vi "FillianProj2.vi"() -> ()   [LabVIEW 2015]
uses:
  <vilib>/Utility/error.llb/Error Cluster From Error Code.vi
  <vilib>/ErrorRing/Error Ring.xnode
panel:
  out "Warnings 2":errorcluster
  out "Current Voltage":dbl(knob) scale=0.0..12.0
  out "Thermometer":dbl(slide) scale=0.0..30.0
  in  "Start/pause":bool
  out "?":bool
  out "?":bool
  out "?":bool
  out "?":bool
  out "?":bool
  out "?":bool
  out "?":bool
  out "?":bool
  out "?":bool
  out "?":bool
  out "?":bool
  out "?":bool
  out "?":bool
  out "?":bool
  out "?":bool
  out "?":bool
  out "Too high":bool
  out "Too low":bool
  out "Too cold":bool
  out "Too hot":bool
  in  "Max temp":sgl(slide) scale=20.0..45.0
  in  "Min temp":sgl(slide) scale=0.0..20.0
  in  "Min voltage":sgl(knob) min=0 max=12 step=0.5 scale=0.0..12.0
  in  "Max voltage":sgl(knob) min=0 max=12 step=0.5 scale=0.0..12.0
  out "Min":dbl(knob) scale=0.0..12.0
  out "Max":dbl(knob) scale=0.0..12.0
  out "Max":dbl(slide) scale=0.0..30.0
  out "Min":dbl(slide) scale=0.0..30.0
  out "Mean":dbl(slide) scale=0.0..30.0
  out "Mean":dbl(knob) scale=0.0..12.0
  out "Voltage":sgl(graph)
  out "Temperature":sgl(graph)
  out "Battery Timeout":bool
  out "Battery Timeout":bool
  out "Link Timeout":bool
  out "Link Timeout":bool
  out "Link Quality":sgl
  out "Battery Voltage":sgl
  out "Battery Voltage":sgl
  out "Link Quality":sgl
  in  "stop 2":bool
  # "Wireless Sensor Network Project"
  # "Temperature Sensor"
  # "Battery"
  # "Link quality"
  # "Voltage Sensor"
  # "Battery"
  # "Link quality"
  # "Warnings"
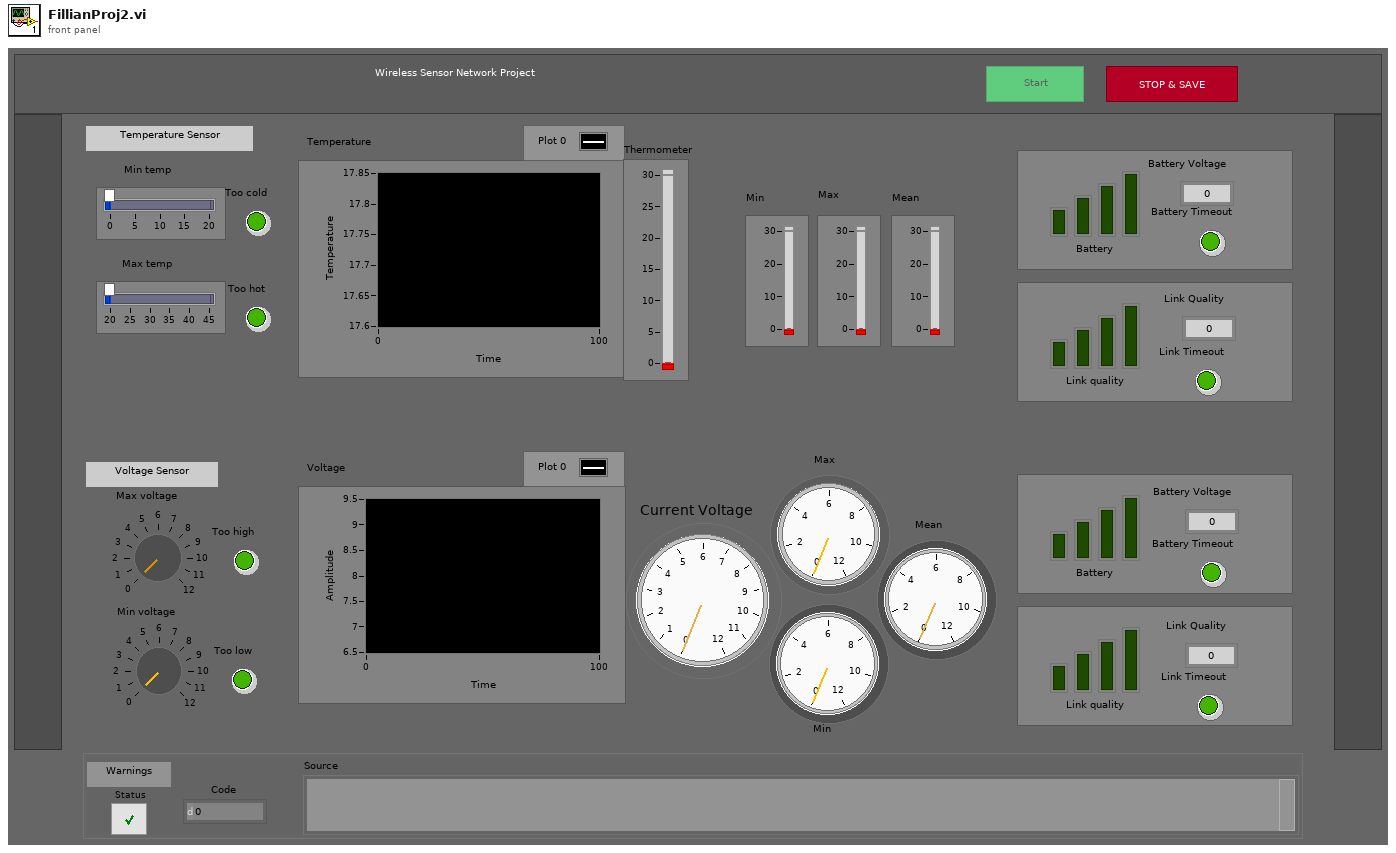
[diagram p1: front panel]
types:
  T1 = enum8{"Enabled", "Disabled", "Disabled and Grayed Out"}
  T2 = enum16{"open", "replace", "create", "open or create", "replace or create", "replace or create with confirmation"}
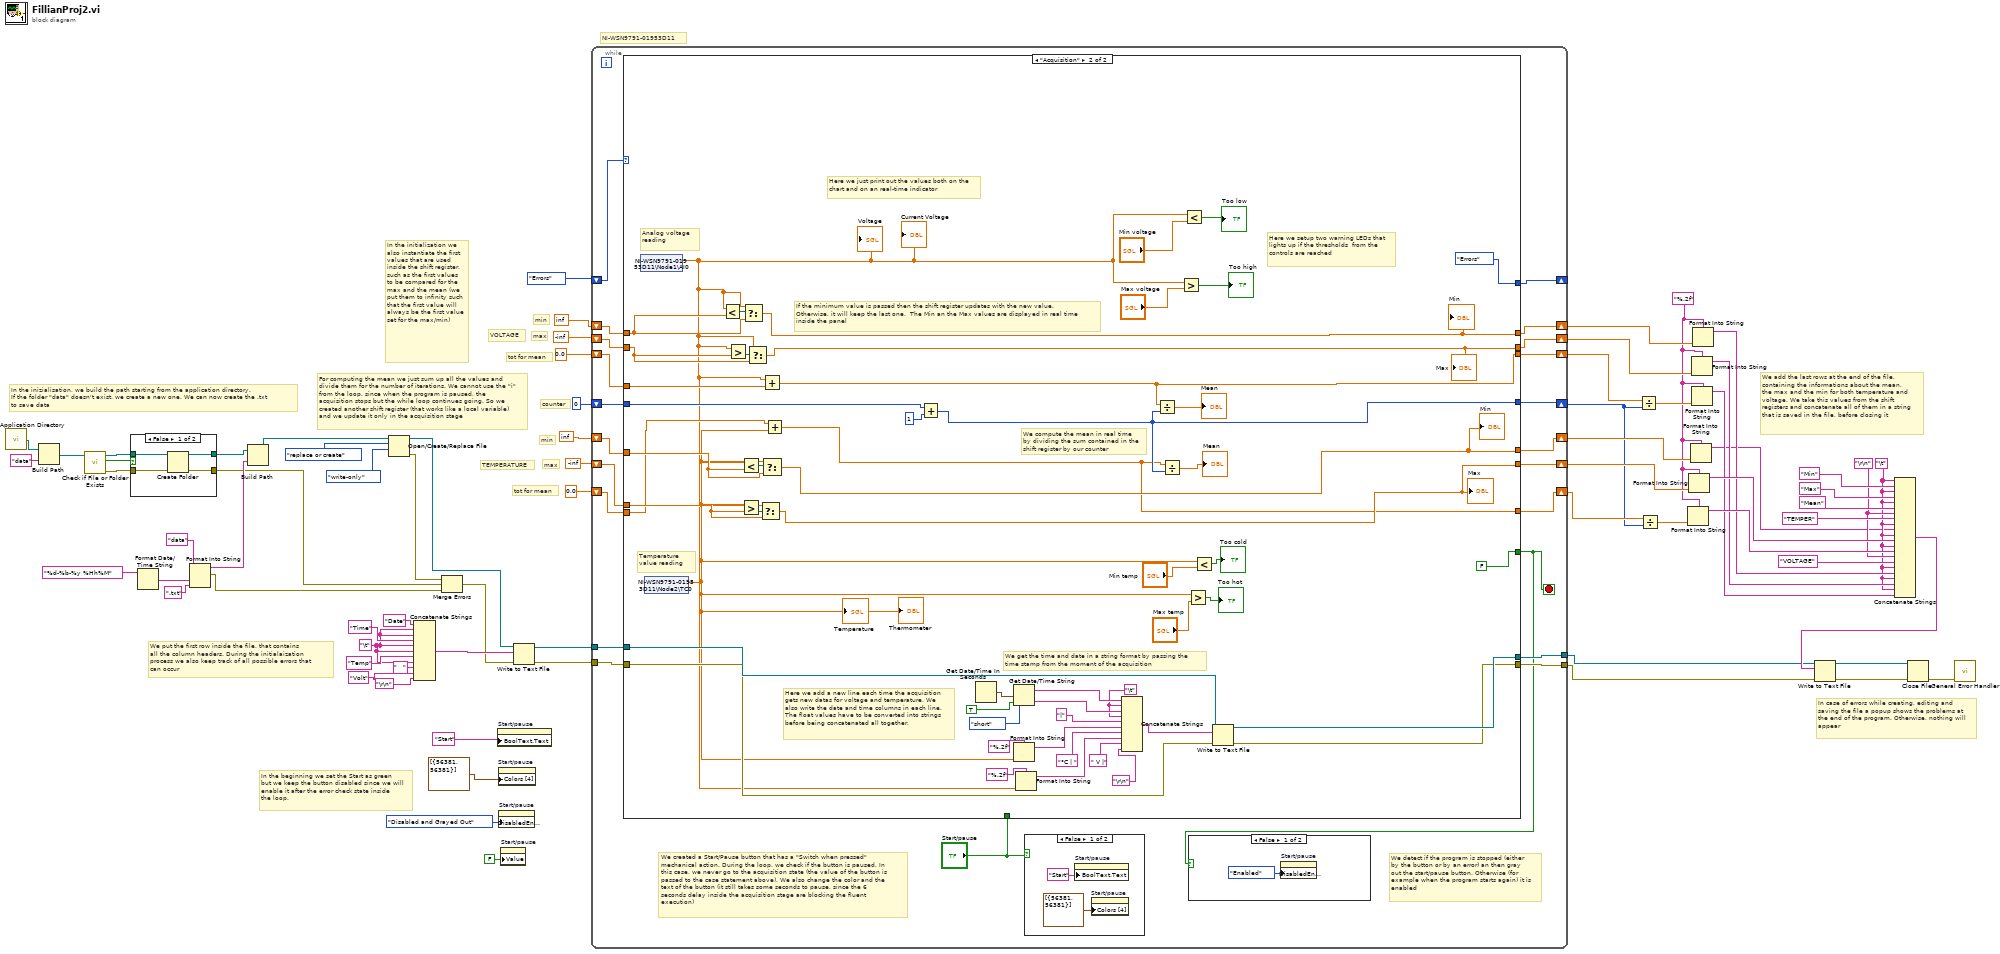
[diagram p0: block diagram]
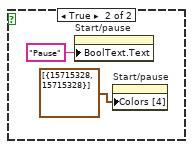
[diagram p3: hidden frame]
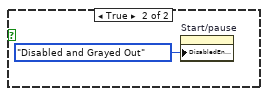
[diagram p4: hidden frame]
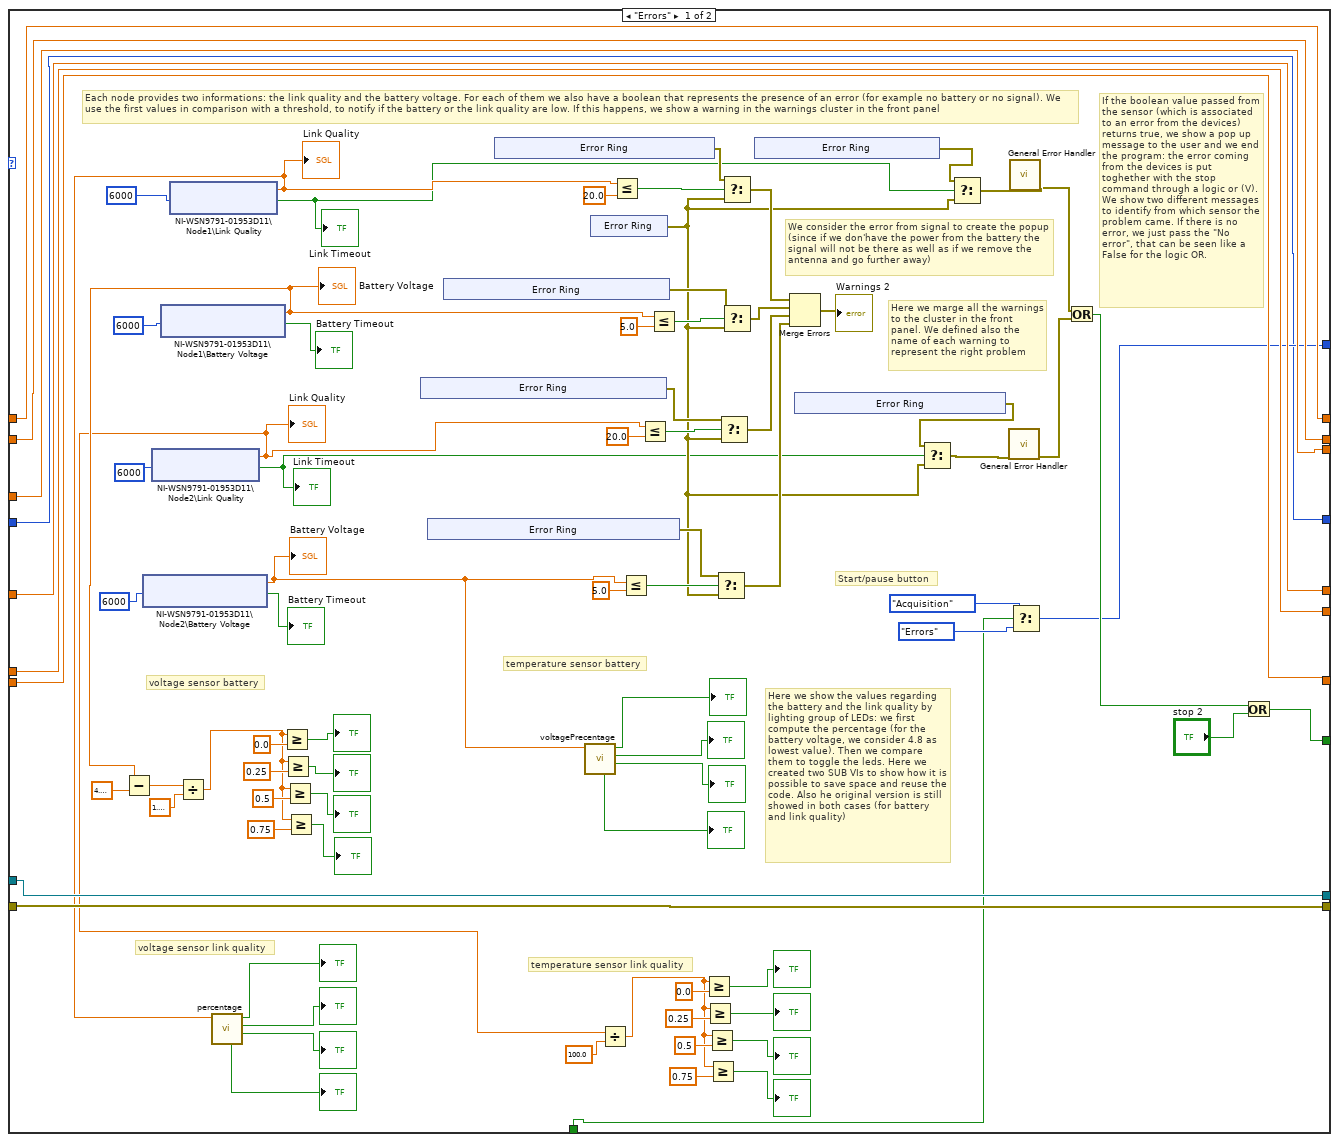
[diagram p5: hidden frame]
diagram:
  w5 = "%.2f" ("format string")
  w22 = "\t"
  w63 = "\r\n"
  w21 = "\t"
  # "We add the last rows at the end of the file, containing the informations about the mean, the max and the min for both temperature and voltage. We take this values from the shift registers and concatenate all of them in a string that is saved in the file, before closing it"
  # "In case of errors while creating, editing and saving the file a popup shows the problems at the end of the program. Otherwise, nothing will appear"
  # "In the beginning we set the Start as green but we keep the button disabled since we will enable it after the error check state inside the loop."
  # "In the initialization we also instantiate the first values that are used inside the shift register, such as the first values to be compared for the max and the mean (we put them to infinity such that the first value will always be the first value set for the max/min)"
  # "We put the first row inside the file, that contains\nall the column headers. During the initialaization \nprocess we also keep track of all possible errors that\ncan occur"
  # "In the inizialisation, we build the path starting from the application directory.\nIf the folder \"data\" doesn't exist, we create a new one. We can now create the .txt \nto save data"
  # "counter"
  # "For computing the mean we just sum up all the values and divide them for the number of iterations. We cannot use the \"i\" from the loop, since when the program is paused, the acquisition stops but the while loop continues going. So we created another shift register (that works like a local variable) and we update it only in the acquisition stage"
  # "NI-WSN9791-01953D11"
  # "max"
  # "tot for mean"
  # "min"
  # "max"
  # "tot for mean"
  # "min"
  # "VOLTAGE"
  # "TEMPERATURE"
  n1 = call <vilib>:"Application Directory.vi"() -> ("Application Directory"=w42:path)
  n2 = Build Path(base path=w42, name or relative path="data") -> (appended path=w40:path)
  n3 = call <vilib>:"Check if File or Folder Exists.vi"("path"=w40) -> ("error out"=w38:errorcluster, "file or folder exists?"=w37:bool, "dup path"=w39:path)  [unwired: 8 in]
  n4 = case shown="False" w37 {
    tunnel: w39 -> [w75 w77]
    tunnel: w38 -> [w74 w76]
    tunnel: [w73 w77] -> w36
    tunnel: [w72 w76] -> w28
    frame False {
      n5 = Create Folder(path (use dialog)=w75, error in=w74) -> (created path=w73:path, error out=w72:errorcluster)  [unwired: 1 in, 1 out]
    }
    frame True {
    }
  }
  n6 = Format Date/Time String(time format string (%c)="%d-%b-%y %Hh%M") -> (date/time string=w33:string)  [unwired: 2 in]
  n7 = Format Into String(initial string="data", w33, ".txt") -> (resulting string=w31:string, error out=w29:errorcluster)  [unwired: 2 in]
  n8 = Build Path(base path=w36, name or relative path=w31) -> (appended path=w30:path)
  n9 = Open/Create/Replace File(file path (use dialog)=w30, operation (0:open)=T2."replace or create", access (0:read/write)=enum16{"read/write", "read-only", "write-only"}."write-only") -> (refnum out=w11:refnum<file>, error out=w12:errorcluster)  [unwired: 3 in, 1 out]
  n10 = Concatenate Strings("Date" ("text"), w22, w22, "Time" ("text"), w22, w22, "Temp" ("text"), w22, "   " ("string"), "Volt" ("text"), "\r\n") -> (w50:string)
  n11 = Merge Errors(w12, w28, w29) -> (w27:errorcluster)
  n12 = property on="Start/pause" class="Bool (strict)"("BoolText.Text"="Start" ("Boolean Text.Text")) -> ()  [unwired: 2 in, 2 out]
  n13 = property on="Start/pause" class="Bool (strict)"("Colors [4]"=cluster{u32, u32}[] [{56381, 56381}]) -> ()  [unwired: 2 in, 2 out]
  n14 = property on="Start/pause" class="Bool (strict)"("DisabledEnum"=T1."Disabled and Grayed Out" ("Disabled")) -> ()  [unwired: 2 in, 2 out]
  n15 = property on="Start/pause" class="Bool (strict)"("Value"=FALSE ("Start/pause")) -> ()  [unwired: 2 in, 2 out]
  n16 = Write to Text File(file (use dialog)=w11, text=w50, error in=w27) -> (refnum out=w48:refnum<file>, error out=w47:errorcluster)  [unwired: 1 in, 1 out]
  n17 = while {
    shift-right: [w93] -> w56
    shift-left: inf -> [w99]
    shift-right: [w92] -> w55
    shift-left: -inf -> [w98]
    shift-right: [w91] -> w44
    shift-left: 0.0 -> [w97]
    shift-right: [w90] -> w54
    shift-left: inf -> [w96]
    shift-right: [w89] -> w53
    shift-left: -inf -> [w95]
    shift-right: [w88] -> w46
    shift-left: 0.0 -> [w94]
    tunnel: [w87] -> w3
    tunnel: [w86] -> w2
    tunnel: w48 -> [w85]
    tunnel: w47 -> [w84]
    shift-right: [w82] -> _
    shift-left: enum16{"Errors", "Acquisition"}."Errors" -> [w83]
    shift-right: [w78] -> w13
    shift-left: 0 -> [w79]
    stop <- w81 stop-if-true
    # "We detect if the program is stopped (either by the button or by an error) an then gray out the start/pause button. Otherwise (for example when the program starts again) it is enabled"
    # "We created a Start/Pause button that has a \"Switch when pressed\" mechanical action. During the loop, we check if the button is paused. In this case, we never go to the acquisition state (the value of the button is passed to the case statement above). We also change the color and the text of the button (it still takes some seconds to pause, since the 6 seconds delay inside the acquisition stage are blocking the fluent execution)"
    n18 = case shown="\"Acquisition\"" w83 {
      tunnel: [w126 enum16{"Errors", "Acquisition"}."Errors"] -> w82
      tunnel: [w109 FALSE] -> w81
      tunnel: w99 -> [w156 w266]
      tunnel: w98 -> [w155 w265]
      tunnel: w97 -> [w154 w264]
      tunnel: w96 -> [w153 w263]
      tunnel: w95 -> [w152 w262]
      tunnel: w94 -> [w151 w224]
      tunnel: [w156 w261] -> w93
      tunnel: [w155 w260] -> w92
      tunnel: [w154 w259] -> w91
      tunnel: [w153 w226] -> w90
      tunnel: [w152 w225] -> w89
      tunnel: [w151 w220] -> w88
      tunnel: [w150 w237] -> w87
      tunnel: [w149 w236] -> w86
      tunnel: w85 -> [w150 w256]
      tunnel: w84 -> [w149 w255]
      tunnel: "Start/pause" -> [w108 _]
      tunnel: w79 -> [w107 w230]
      tunnel: [w107 w229] -> w78
      frame "Errors" {
        # "Here we show the values regarding the battery and the link quality by lighting group of LEDs: we first compute the percentage (for the battery voltage, we consider 4.8 as lowest value). Then we compare them to toggle the leds. Here we created two SUB VIs to show how it is possible to save space and reuse the code. Also he original version is still showed in both cases (for battery and link quality)"
        # "Here we marge all the warnings to the cluster in the front panel. We defined also the name of each warning to represent the right problem"
        # "We consider the error from signal to create the popup (since if we don'have the power from the battery the signal will not be there as well as if we remove the antenna and go further away)"
        # "If the boolean value passed from the sensor (which is associated to an error from the devices) returns true, we show a pop up message to the user and we end the program: the error coming from the devices is put toghether with the stop command through a logic or (V). We show two different messages to identify from which sensor the problem came. If there is no error, we just pass the \"No error\", that can be seen like a False for the logic OR."
        # "Each node provides two informations: the link quality and the battery voltage. For each of them we also have a boolean that represents the presence of an error (for example no battery or no signal). We use the first values in comparison with a threshold, to notify if the battery or the link quality are low. If this happens, we show a warning in the warnings cluster in the front panel"
        # "temperature sensor link quality"
        # "voltage sensor link quality"
        # "temperature sensor battery"
        # "voltage sensor battery"
        # "Start/pause button"
        n19 = shared-variable "NI-WSN9791-01953D11\\Node2\\Battery Voltage"(6000 ("ms timeout (0)")) -> (w148:sgl, →"Battery Timeout":bool)  [unwired: 1 in, 1 out]
        "Battery Voltage" <- w148
        n20 = shared-variable "NI-WSN9791-01953D11\\Node2\\Link Quality"(6000 ("ms timeout (0)")) -> (w110:sgl, w129:bool)  [unwired: 1 in, 1 out]
        "Link Quality" <- w110
        "Link Timeout" <- w129
        n21 = shared-variable "NI-WSN9791-01953D11\\Node1\\Battery Voltage"(6000 ("ms timeout (0)")) -> (w131:sgl, →"Battery Timeout":bool)  [unwired: 1 in, 1 out]
        "Battery Voltage" <- w131
        n22 = Subtract(x=w131, y=sgl 4.8) -> (x-y=w142:sgl)
        n23 = shared-variable "NI-WSN9791-01953D11\\Node1\\Link Quality"(6000 ("ms timeout (0)")) -> (w121:sgl, w106:bool)  [unwired: 1 in, 1 out]
        "Link Quality" <- w121
        "Link Timeout" <- w106
        n24 = Divide(x=w142, y=sgl 1.4) -> (x/y=w136:sgl)
        n25 = call "percentage.vi"("Numeric"=w121) -> ("Boolean 2"=→"?":bool, "Boolean 3"=→"?":bool, "Boolean 4"=→"?":bool, "Boolean"=→"?":bool)  [unwired: 7 in]
        n26 = Greater Or Equal?(x=w136, y=0.0) -> (x >= y?=→"?":bool)
        n27 = Greater Or Equal?(x=w136, y=0.25) -> (x >= y?=→"?":bool)
        n28 = Greater Or Equal?(x=w136, y=0.5) -> (x >= y?=→"?":bool)
        n29 = Greater Or Equal?(x=w136, y=0.75) -> (x >= y?=→"?":bool)
        n30 = xnode "Error Ring"() -> ("error out"=w184:errorcluster)
        n31 = xnode "Error Ring"() -> ("error out"=w172:errorcluster)
        n32 = xnode "Error Ring"() -> ("error out"=w179:errorcluster)
        n33 = xnode "Error Ring"() -> ("error out"=w181:errorcluster)
        n34 = call "voltagePrecentage.vi"("Numeric"=w148) -> ("Boolean 2"=→"?":bool, "Boolean 3"=→"?":bool, "Boolean 4"=→"?":bool, "Boolean"=→"?":bool)  [unwired: 7 in]
        n35 = xnode "Error Ring"() -> ("error out"=w162:errorcluster)
        n36 = Divide(x=w110, y=sgl 100.0) -> (x/y=w115:sgl)
        n37 = Less Or Equal?(x=w121, y=sgl 20.0) -> (x <= y?=w182:bool)
        n38 = Less Or Equal?(x=w148, y=sgl 5.0) -> (x <= y?=w173:bool)
        n39 = Less Or Equal?(x=w110, y=sgl 20.0) -> (x <= y?=w185:bool)
        n40 = Less Or Equal?(x=w131, y=sgl 5.0) -> (x <= y?=w180:bool)
        n41 = Greater Or Equal?(x=w115, y=0.0) -> (x >= y?=→"?":bool)
        n42 = Greater Or Equal?(x=w115, y=0.25) -> (x >= y?=→"?":bool)
        n43 = Greater Or Equal?(x=w115, y=0.5) -> (x >= y?=→"?":bool)
        n44 = Greater Or Equal?(x=w115, y=0.75) -> (x >= y?=→"?":bool)
        n45 = Select(t=w172, s=w173, f=w162) -> (s? t:f=w171:errorcluster)
        n46 = Select(t=w184, s=w185, f=w162) -> (s? t:f=w175:errorcluster)
        n47 = Select(t=w181, s=w182, f=w162) -> (s? t:f=w177:errorcluster)
        n48 = Select(t=w179, s=w180, f=w162) -> (s? t:f=w178:errorcluster)
        n49 = xnode "Error Ring"() -> ("error out"=w164:errorcluster)
        n50 = Merge Errors(w177, w178, w175, w171) -> (→"Warnings 2":errorcluster)
        n51 = xnode "Error Ring"() -> ("error out"=w163:errorcluster)
        n52 = Select(t=w163, s=w129, f=w162) -> (s? t:f=w160:errorcluster)
        n53 = Select(t=w164, s=w106, f=w162) -> (s? t:f=w161:errorcluster)
        n54 = call <vilib>:"General Error Handler.vi"("error in (no error)"=w160) -> ("error out"=w158:errorcluster)  [unwired: 10 in, 4 out]
        n55 = call <vilib>:"General Error Handler.vi"("error in (no error)"=w161) -> ("error out"=w159:errorcluster)  [unwired: 10 in, 4 out]
        n56 = Select(t=enum16{"Errors", "Acquisition"}."Acquisition", s=w108, f=enum16{"Errors", "Acquisition"}."Errors") -> (s? t:f=w126:enum16{"Errors", "Acquisition"})
        n57 = Or(x=w159, y=w158) -> (x .or. y?=w157:bool)
        n58 = Or(x=w157, y="stop 2") -> (x .or. y?=w109:bool)
      }
      frame "Acquisition" {
        w241 = "\t"
        # "We compute the mean in real time by dividing the sum contained in the shift register by our counter"
        # "We get the time and date in a string format by passing the time stamp from the moment of the acquisition"
        # "Here we add a new line each time the acquisition gets new datas for voltage and temperature. We also write the date and time columns in each line. The float values have to be converted into strings before being concatenated all together."
        # "If the minimum value is passed then the shift register updates with the new value. Otherwise, it will keep the last one.  The Min an the Max values are displayed in real time inside the panel"
        # "Here we setup two warning LEDs that lights up if the thresholds  from the controls are reached"
        # "Here we just print out the values both on the chart and on an real-time indicator"
        # "Analog voltage reading"
        # "Temperature value reading"
        n59 = shared-variable "NI-WSN9791-01953D11\\Node1\\AI0"() -> (w223:sgl)  [unwired: 1 in, 1 out]
        "Voltage" <- w223
        "Current Voltage" <- w223
        n60 = shared-variable "NI-WSN9791-01953D11\\Node2\\TC0"() -> (w222:sgl)  [unwired: 1 in, 1 out]
        "Temperature" <- w222
        "Thermometer" <- w222
        n61 = Less?(x=w223, y=w266) -> (x < y?=w269:bool)
        n62 = Greater?(x=w223, y=w265) -> (0:w270:bool)
        n63 = Less?(x=w222, y=w263) -> (x < y?=w268:bool)
        n64 = Greater?(x=w222, y=w262) -> (0:w267:bool)
        n65 = Select(t=w223, s=w269, f=w266) -> (s? t:f=w261:dbl)
        "Min" <- w261
        n66 = Select(t=w223, s=w270, f=w265) -> (s? t:f=w260:dbl)
        "Max" <- w260
        n67 = Select(t=w222, s=w267, f=w262) -> (s? t:f=w225:dbl)
        "Max" <- w225
        n68 = Add(x=w223, y=w264) -> (x+y=w259:dbl)
        n69 = Select(t=w222, s=w268, f=w263) -> (s? t:f=w226:dbl)
        "Min" <- w226
        n70 = Add(x=w224, y=w222) -> (x+y=w220:dbl)
        n71 = Add(x=w230, y=1) -> (x+y=w229:i32)
        n72 = Get Date/Time In Seconds() -> (seconds since 1Jan1904=w221:timestamp)
        n73 = Get Date/Time String(date format (0)=enum16{"short", "long", "abbreviated"}."short", seconds (now)=w221, want seconds? (F)=TRUE) -> (date string=w243:string, time string=w242:string)
        n74 = Format Into String(format string="%.2f", w222) -> (resulting string=w234:string)  [unwired: 2 in, 1 out]
        n75 = Format Into String(format string="%.2f", w223) -> (resulting string=w232:string)  [unwired: 2 in, 1 out]
        n76 = Concatenate Strings(w243, w241, w242, w241, "|" ("string"), w234, "°C | " ("string"), w232, " V |" ("string"), "\r\n") -> (w227:string)
        n77 = Divide(x=w259, y=w229) -> (x/y=→"Mean":dbl)
        n78 = Divide(x=w220, y=w229) -> (x/y=→"Mean":dbl)
        n79 = Greater?(x=w223, y="Max voltage") -> (0:→"Too high":bool)
        n80 = Less?(x=w223, y="Min voltage") -> (x < y?=→"Too low":bool)
        n81 = Greater?(x=w222, y="Max temp") -> (0:→"Too hot":bool)
        n82 = Less?(x=w222, y="Min temp") -> (x < y?=→"Too cold":bool)
        n83 = Write to Text File(file (use dialog)=w256, text=w227, error in=w255) -> (refnum out=w237:refnum<file>, error out=w236:errorcluster)  [unwired: 1 in, 1 out]
      }
    }
    n84 = case shown="False" "Start/pause" {
      frame False {
        n85 = property on="Start/pause" class="Bool (strict)"("BoolText.Text"="Start" ("Boolean Text.Text")) -> ()  [unwired: 2 in, 2 out]
        n86 = property on="Start/pause" class="Bool (strict)"("Colors [4]"=cluster{u32, u32}[] [{56381, 56381}]) -> ()  [unwired: 2 in, 2 out]
      }
      frame True {
        n87 = property on="Start/pause" class="Bool (strict)"("BoolText.Text"="Pause" ("Boolean Text.Text")) -> ()  [unwired: 2 in, 2 out]
        n88 = property on="Start/pause" class="Bool (strict)"("Colors [4]"=cluster{u32, u32}[] [{15715328, 15715328}]) -> ()  [unwired: 2 in, 2 out]
      }
    }
    n89 = case shown="False" w81 {
      frame False {
        n90 = property on="Start/pause" class="Bool (strict)"("DisabledEnum"=T1."Enabled" ("Disabled")) -> ()  [unwired: 2 in, 2 out]
      }
      frame True {
        n91 = property on="Start/pause" class="Bool (strict)"("DisabledEnum"=T1."Disabled and Grayed Out" ("Disabled")) -> ()  [unwired: 2 in, 2 out]
      }
    }
  }
  n92 = Divide(x=w44, y=w13) -> (x/y=w43:dbl)
  n93 = Divide(x=w46, y=w13) -> (x/y=w45:dbl)
  n94 = Format Into String(format string=w5, w45) -> (resulting string=w64:string)  [unwired: 2 in, 1 out]
  n95 = Format Into String(format string=w5, w53) -> (resulting string=w65:string)  [unwired: 2 in, 1 out]
  n96 = Format Into String(format string=w5, w54) -> (resulting string=w4:string)  [unwired: 2 in, 1 out]
  n97 = Format Into String(format string=w5, w55) -> (resulting string=w60:string)  [unwired: 2 in, 1 out]
  n98 = Format Into String(format string=w5, w43) -> (resulting string=w59:string)  [unwired: 2 in, 1 out]
  n99 = Format Into String(format string=w5, w56) -> (resulting string=w61:string)  [unwired: 2 in, 1 out]
  n100 = Concatenate Strings(w21, "Min", w21, "Max", w21, "Mean", w63, "TEMPER", w21, w4, w21, w65, w21, w64, w63, "VOLTAGE", w21, w61, w21, w60, w21, w59) -> (w58:string)
  n101 = Write to Text File(file (use dialog)=w3, text=w58, error in=w2) -> (refnum out=w57:refnum<file>, error out=w1:errorcluster)  [unwired: 1 in, 1 out]
  n102 = Close File(refnum=w57, error in=w1) -> (error out=w10:errorcluster)  [unwired: 1 out]
  n103 = call <vilib>:"General Error Handler.vi"("error in (no error)"=w10) -> ()  [unwired: 10 in, 5 out]
